vi "Calibrate Camera.vi"(5 "Termination Criteria (Default: Default Criteria)":refnum<class "Termination Criteria.lvclass">, 6 "Camera Parameters (Estimate)":T13, 7 "Flags (Default: Empty)":T4[](array[typedef]), 8 "error in (no error)":errorcluster, 9 "Fixed Point Index (Default -1: Do not use RO mode)":i32=-1, 10 "Image Size":T12={"Width"=1920, "Height"=1080}, 11 "Point Correspondences":T5) -> (0 "error out":errorcluster, 1 "RMS Error":dbl[](array[numeric]), 3 "Camera Parameters":T9, 4 "Poses":T1[](array[typedef]))   [LabVIEW 2020, in "g_ar_toolkit.ar.lvlib"]
uses:
  g_ar_toolkit.ar.lvlib
  Camera Parameters Estimate.ctl
  g_ar_toolkit.common/Camera Matrix.ctl
  g_ar_toolkit.common/Camera Distortion Coefficients.ctl
  g_ar_toolkit.common/Image Size (Integer).ctl
  g_ar_toolkit.common/Camera Parameters.ctl
  Point Correspondence Sets.ctl
  Point Correspondence Set.ctl
  g_ar_toolkit.common/Object Point (Float).ctl
  g_ar_toolkit.common/Image Point (Float).ctl
  Camera Calibration Flags.ctl
  g_ar_toolkit.common/Termination Criteria/Termination Criteria.lvclass
  Pose.ctl
  rvec.ctl
  g_ar_toolkit.common/tvec.ctl
  g_ar_toolkit.common/Termination Criteria/Termination Criteria.lvclass/Termination Criteria.ctl
  g_ar_toolkit.common/g_ar_toolkit.common.lvlib
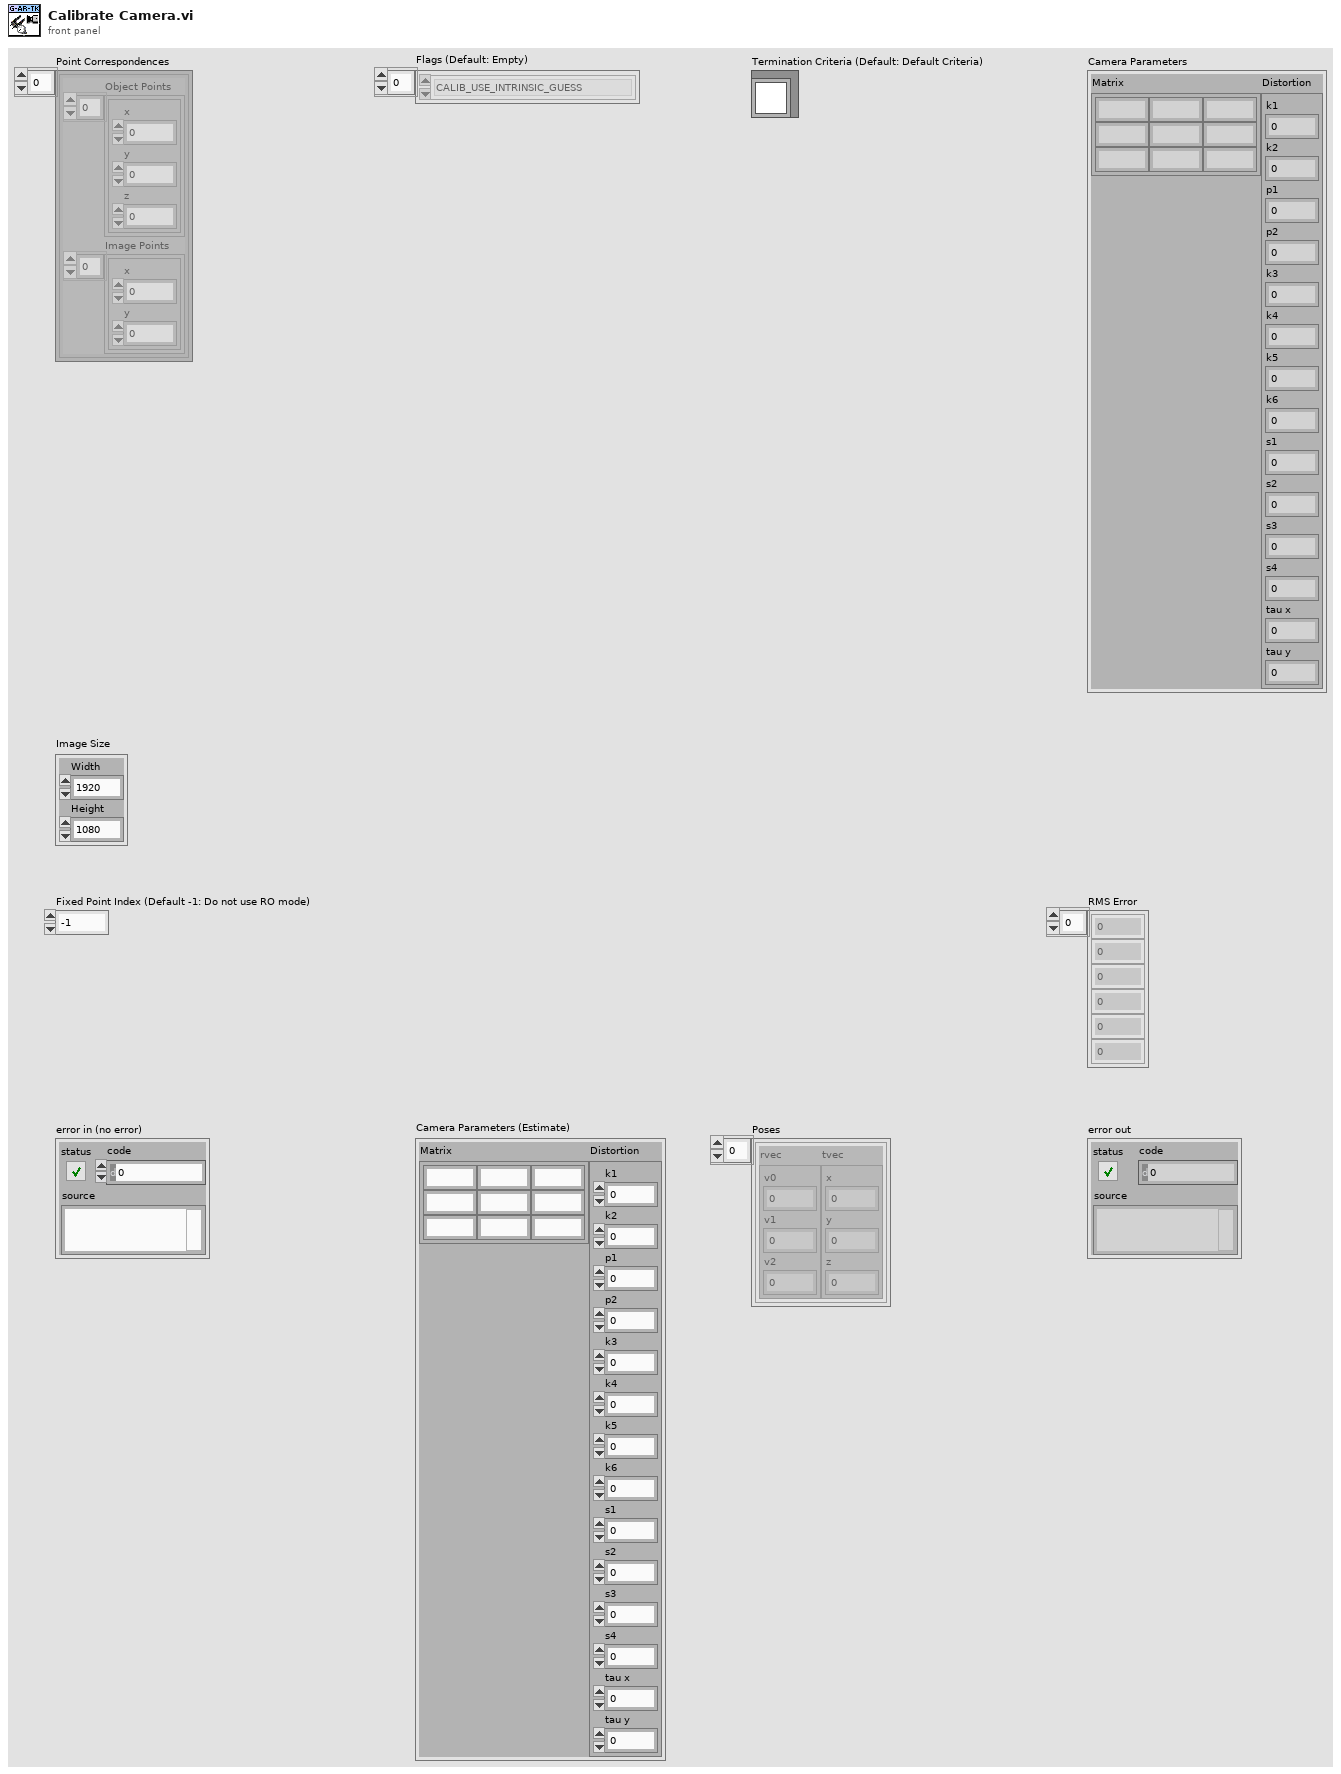
[diagram p1: front panel]
types:
  T1 = typedef "g_ar_toolkit.ar.lvlib/Pose.ctl" = cluster{"rvec":T2, "tvec":T3}
  T2 = typedef "g_ar_toolkit.ar.lvlib/rvec.ctl" = cluster{"v0":dbl, "v1":dbl, "v2":dbl}
  T3 = typedef "g_ar_toolkit.ar.lvlib/tvec.ctl" = cluster{"x":dbl, "y":dbl, "z":dbl}
  T4 = typedef "g_ar_toolkit.ar.lvlib/Camera Calibration Flags.ctl" = enum16{"CALIB_USE_INTRINSIC_GUESS", "CALIB_FIX_PRINCIPAL_POINT", "CALIB_FIX_ASPECT_RATIO", "CALIB_ZERO_TANGENT_DIST", "CALIB_FIX_FOCAL_LENGTH", "CALIB_FIX_K1", "CALIB_RATIONAL_MODEL", "CALIB_THIN_PRISM_MODEL", "CALIB_FIX_S1_S2_S3_S4", "CALIB_TILTED_MODEL", "CALIB_FIX_TAUX_TAUY"}
  T5 = typedef "g_ar_toolkit.ar.lvlib/Point Correspondence Sets.ctl" = T6[]
  T6 = typedef "g_ar_toolkit.ar.lvlib/Point Correspondence Set.ctl" = cluster{"Object Points":T7[], "Image Points":T8[]}
  T7 = typedef "g_ar_toolkit.common.lvlib/Object Point (Float).ctl" = cluster{"x":dbl, "y":dbl, "z":dbl}
  T8 = typedef "g_ar_toolkit.common.lvlib/Image Point (Float).ctl" = cluster{"x":dbl, "y":dbl}
  T9 = typedef "g_ar_toolkit.common.lvlib/Camera Parameters.ctl" = cluster{"Matrix":T10, "Distortion":T11}
  T10 = typedef "g_ar_toolkit.common.lvlib/Camera Matrix.ctl" = cluster{"m 0,0":dbl, "m 0,1":dbl, "m 0,2":dbl, "m 1,0":dbl, "m 1,1":dbl, "m 1,2":dbl, "m 2,0":dbl, "m 2,1":dbl, "m 2,2":dbl}
  T11 = typedef "g_ar_toolkit.common.lvlib/Camera Distortion Coefficients.ctl" = cluster{"k1":dbl, "k2":dbl, "p1":dbl, "p2":dbl, "k3":dbl, "k4":dbl, "k5":dbl, "k6":dbl, "s1":dbl, "s2":dbl, "s3":dbl, "s4":dbl, "tau x":dbl, "tau y":dbl}
  T12 = typedef "g_ar_toolkit.common.lvlib/Image Size (Integer).ctl" = cluster{"Width":u16, "Height":u16}
  T13 = typedef "g_ar_toolkit.ar.lvlib/Camera Parameters Estimate.ctl" = cluster{"Matrix":T10, "Distortion":T11}
  T14 = typedef "g_ar_toolkit.common.lvlib/Termination Criteria.lvclass/Termination Criteria Values.ctl" = cluster{"Epsilon":dbl, "Iterations":i32}
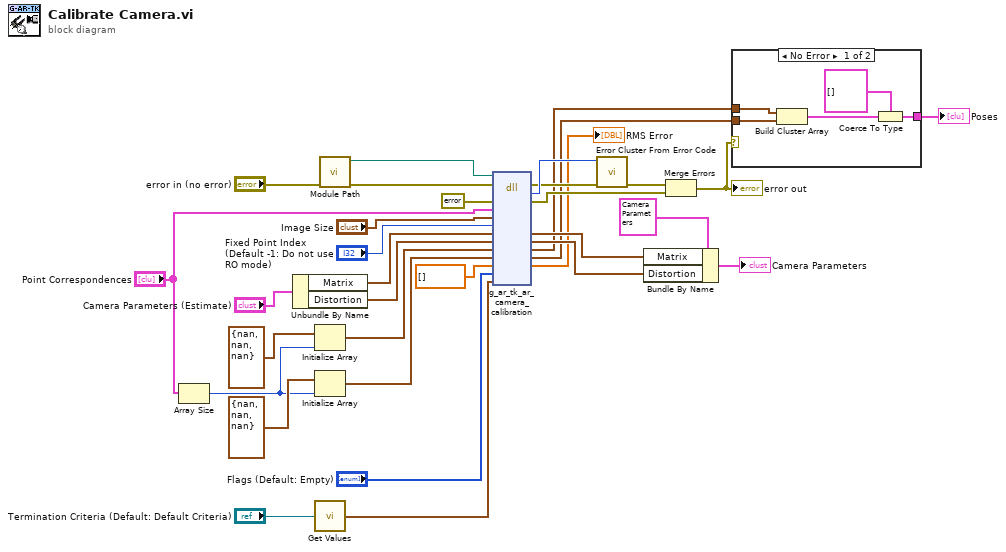
[diagram p0: block diagram]
diagram:
  n1 = Array Size(array="Point Correspondences") -> (size(s)=w12:i32)
  n2 = Unbundle By Name("Camera Parameters (Estimate)") -> ("Matrix"=w20:T10, "Distortion"=w19:T11)
  n3 = Initialize Array(T2 {"v0"=nan, "v1"=nan, "v2"=nan} ("rvec"), w12) -> (w23:T2[])
  n4 = Initialize Array(T3 {"x"=nan, "y"=nan, "z"=nan} ("tvec"), w12) -> (w21:T3[])
  n5 = call "Get Values.vi"("Termination Criteria in"="Termination Criteria (Default: Default Criteria)") -> ("Term Criteria"=w5:T14)
  n6 = call "Module Path.vi"("error in (no error)"="error in (no error)") -> ("error out"=w2:errorcluster, "Path"=w1:path)  [unwired: 9 in]
  n7 = dll-call lib="?" fn="g_ar_tk_ar_camera_calibration" ("g_ar_toolkit.*.*:g_ar_tk_image_copy")(path in=w1, error in=w2, "error_cluster"=errorcluster {"status"=FALSE, "code"=0, "source"=""} ("error constant"), "corespondences"="Point Correspondences", "image_size"="Image Size", "fixed_point"="Fixed Point Index (Default -1: Do not use RO mode)", "camera_matrix"=w20, "camera_distortion"=w19, "rvecs"=w23, "tvecs"=w21, "rms_errors"=dbl[] [], "flags"="Flags (Default: Empty)", "termination_crit"=w5) -> (error out=w27:errorcluster, "MgErr"=w28:i32, "error_cluster"=w31:errorcluster, "camera_matrix"=w18:T10, "camera_distortion"=w17:T11, "rvecs"=w15:T2[], "tvecs"=w14:T3[], "rms_errors"=→"RMS Error":dbl[])  [unwired: 6 in, 1 out]
  n8 = call <vilib>:"Error Cluster From Error Code.vi"("error in (no error)"=w27, "error code (0)"=w28) -> ("error out"=w29:errorcluster)  [unwired: 7 in]
  n9 = Bundle By Name(cluster=T9 {"Matrix"={"m 0,0"=0.0, "m 0,1"=0.0, "m 0,2"=0.0, "m 1,0"=0.0, "m 1,1"=0.0, "m 1,2"=0.0, "m 2,0"=0.0, "m 2,1"=0.0, "m 2,2"=0.0}, "Distortion"={"k1"=0.0, "k2"=0.0, "p1"=0.0, "p2"=0.0, "k3"=0.0, "k4"=0.0, "k5"=0.0, "k6"=0.0, "s1"=0.0, "s2"=0.0, "s3"=0.0, "s4"=0.0, "tau x"=0.0, "tau y"=0.0}} ("Camera Parameters"), "Matrix"=w18, "Distortion"=w17) -> (→"Camera Parameters":T9)
  n10 = Merge Errors(w29, w31) -> (w11:errorcluster)
  "error out" <- w11
  n11 = case shown="No Error" w11 {
    tunnel: w15 -> [w37 _]
    tunnel: w14 -> [w36 _]
    tunnel: [w33 _] -> w13
    frame No Error {
      n12 = Build Cluster Array(w37, w36) -> (w34:cluster{"rvec":T2, "tvec":T3}[])
      n13 = Coerce To Type(0:w34, 1:T1[] [] ("Array")) -> (2:w33:T1[])
    }
    frame Error {
    }
  }
  "Poses" <- w13
